vi "Set_IstanceName.vi"(8 "error in (no error)":errorcluster, 10 "IstanceName":string, 11 "ObserverClass in":refnum<class "ObserverClass.lvclass">) -> (0 "error out":errorcluster, 3 "ObserverClass out":refnum<class "ObserverClass.lvclass">)   [LabVIEW 2025, in "ObserverClass.lvlib" / "ObserverClass.lvclass"]
uses:
  ObserverClass.lvclass
  ObserverClass.lvclass/ObserverClass.ctl
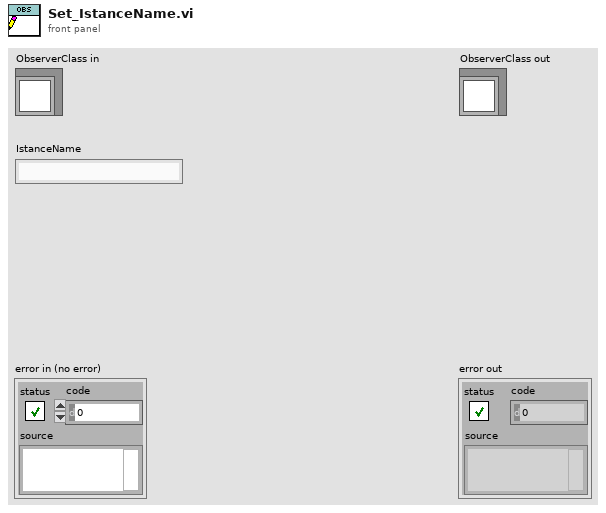
[diagram p1: front panel]
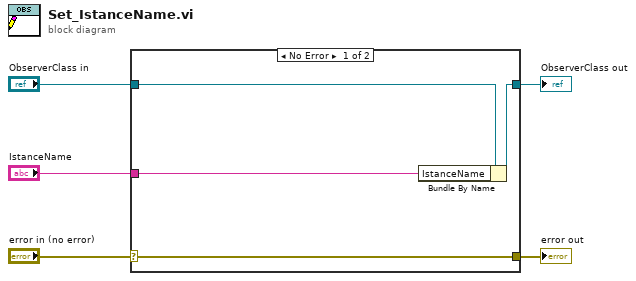
[diagram p0: block diagram]
diagram:
  n1 = case shown="No Error" "error in (no error)" {
    selector: "error in (no error)" -> [w9 w10]
    tunnel: [w9 w10] -> w4
    tunnel: [w7 w11] -> w2
    tunnel: "ObserverClass in" -> [w8 w11]
    tunnel: "IstanceName" -> [w6 _]
    frame No Error {
      n2 = Bundle By Name(cluster=w8, "IstanceName"=w6) -> (w7:refnum<class "ObserverClass.lvclass">)
    }
    frame Error {
    }
  }
  "error out" <- w4
  "ObserverClass out" <- w2
